vi "unique parent class name.vi"(11 "class name":string) -> (3 "String":string)   [LabVIEW 2020, in "Publisher Subscriber.lvlib"]
uses:
  Publisher Subscriber.lvlib
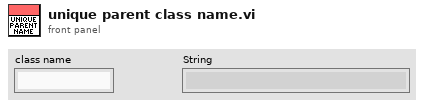
[diagram p1: front panel]
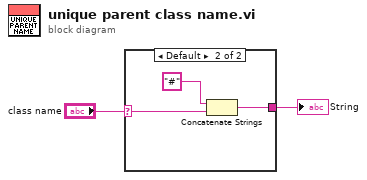
[diagram p0: block diagram]
diagram:
  n1 = case shown="Default" "class name" {
    selector: "class name" -> [_ w3]
    tunnel: [_ w5] -> w2
    frame "LabVIEW Object" {
    }
    frame Default {
      n2 = Concatenate Strings("#" ("string"), w3) -> (w5:string)
    }
  }
  "String" <- w2
